vi "Build_DTU_Info_LS1.vi"(8 "error in":errorcluster caption="entrée d'erreur (pas d'erreur)", 11 "DescKword":string) -> (0 "error out":errorcluster caption="sortie d'erreur", 1 "ScanParUser":string, 2 "ScanParTime":string, 3 "ScanParDate":string, 4 "DTU_HdrStr":string, 5 "FileNmDTString":string)   [LabVIEW 2019]
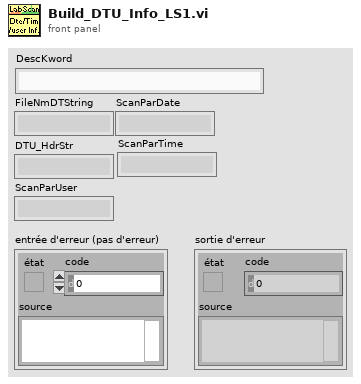
[diagram p1: front panel]
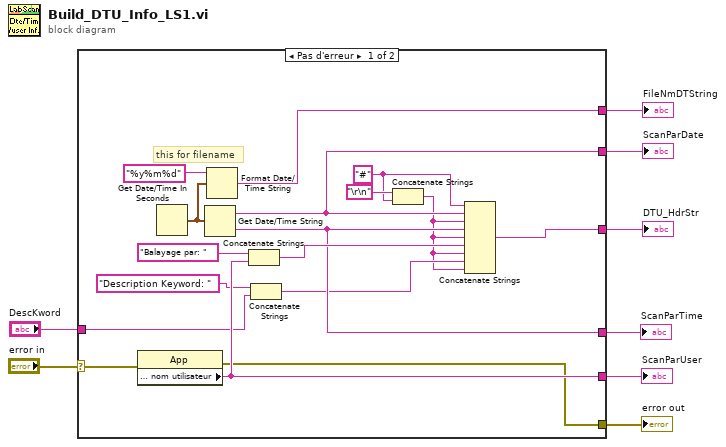
[diagram p0: block diagram]
diagram:
  n1 = case shown="Pas d'erreur" "error in" {
    selector: "error in" -> [w14 w26]
    tunnel: [w21 _] -> w8
    tunnel: [w19 _] -> w7
    tunnel: [w17 _] -> w6
    tunnel: [w16 _] -> w5
    tunnel: [w15 _] -> w4
    tunnel: [w13 w26] -> w2
    tunnel: "DescKword" -> [w11 _]
    frame No Error {
      w24 = "#" ("chaîne")
      # "this for filename"
      n2 = property class="App"(error in=w14) -> (error out=w13:errorcluster, "Application : nom utilisateur"=w15:string)  [unwired: 1 in, 1 out]
      n3 = Get Date/Time In Seconds() -> (seconds since 1Jan1904=w22:timestamp)
      n4 = Get Date/Time String(seconds (now)=w22) -> (date string=w21:string, time string=w16:string)  [unwired: 2 in]
      n5 = Format Date/Time String(time format string (%c)="%y%m%d" ("chaîne de format de l'heure (%c)"), seconds (now)=w22) -> (date/time string=w19:string)  [unwired: 1 in]
      n6 = Concatenate Strings("Balayage par: " ("string"), w15) -> (w18:string)
      n7 = Concatenate Strings("Description Keyword: " ("string"), w11) -> (w10:string)
      n8 = Concatenate Strings("\r\n", w24) -> (w9:string)
      n9 = Concatenate Strings(w24, w21, w9, w16, w9, w18, w9, w10, w9) -> (w17:string)
    }
    frame Error {
    }
  }
  "FileNmDTString" <- w7
  "DTU_HdrStr" <- w6
  "ScanParDate" <- w8
  "ScanParTime" <- w5
  "ScanParUser" <- w4
  "error out" <- w2
